vi "Subtract Resources (SubVI).vi"(8 "error in (no error)":errorcluster, 10 "Simulation in":cluster{"Water":dbl, "Coffee":dbl, "Milk":dbl}, 11 "Coffee Selection":T1) -> (0 "error out":errorcluster, 2 "Simulation out":cluster{"Water":dbl, "Coffee":dbl, "Milk":dbl}, 3 "Coffe and Chamber increase":cluster{"coffee":i8, "chamber":i8})   [LabVIEW 2017]
panel:
  # "input values"
  # "output values"
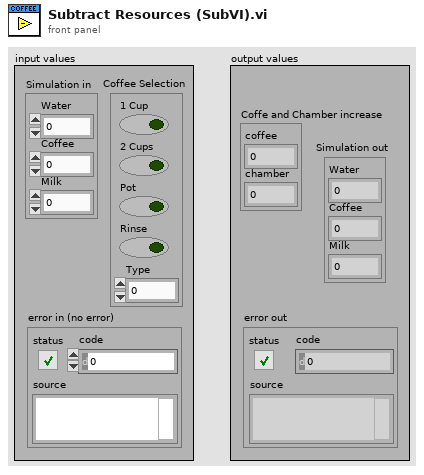
[diagram p1: front panel]
types:
  T1 = cluster{"1 Cup":bool, "2 Cups":bool, "Pot":bool, "Rinse":bool, "Type":i8}
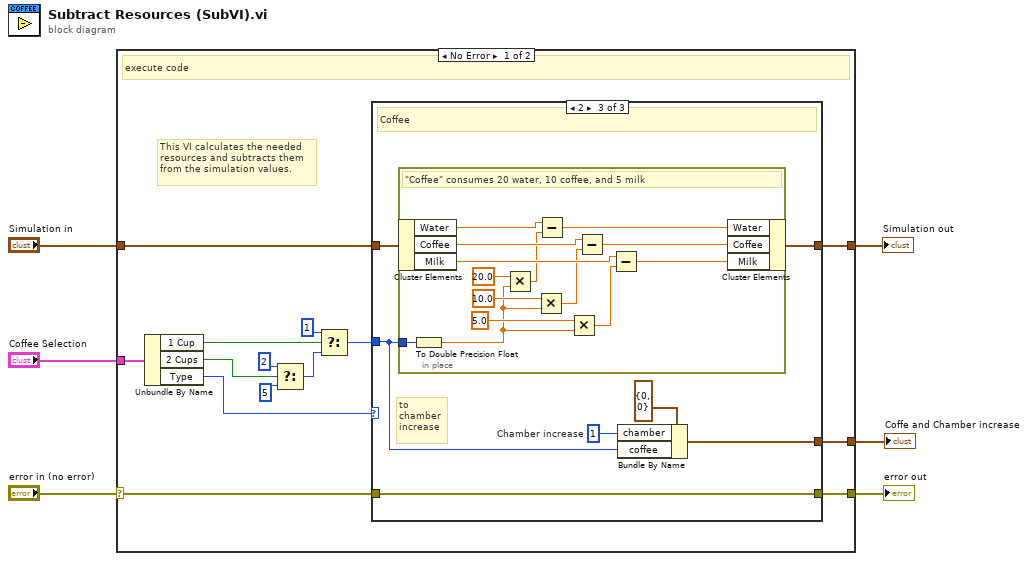
[diagram p0: block diagram]
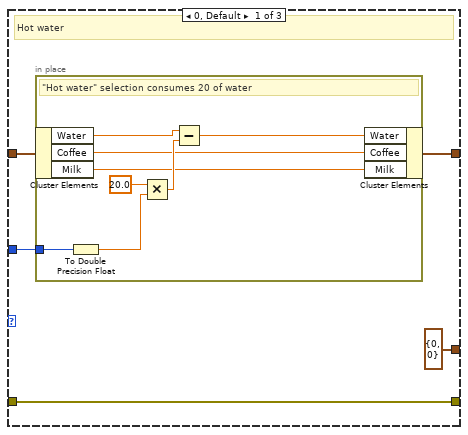
[diagram p2: hidden frame]
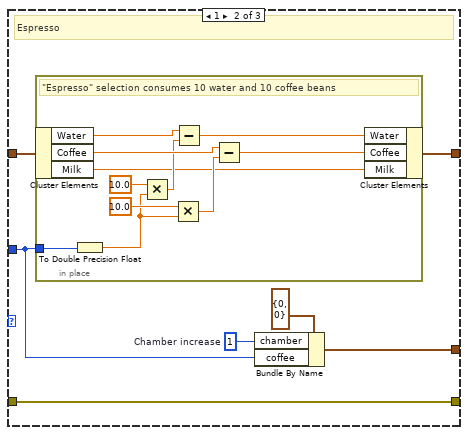
[diagram p3: hidden frame]
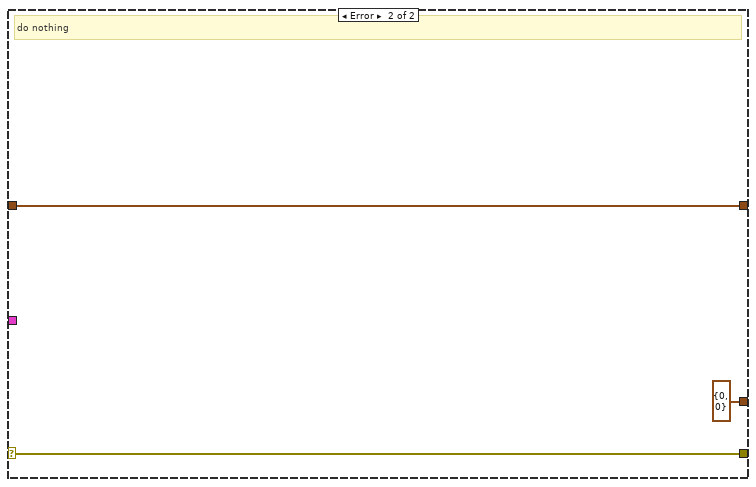
[diagram p4: hidden frame]
diagram:
  n1 = case shown="No Error" "error in (no error)" {
    selector: "error in (no error)" -> [w17 w74]
    tunnel: "Simulation in" -> [w20 w75]
    tunnel: "Coffee Selection" -> [w19 _]
    tunnel: [w18 w75] -> w4
    tunnel: [w16 w74] -> w2
    tunnel: [w15 cluster{"coffee":i8, "chamber":i8} {"coffee"=0, "chamber"=0} ("input cluster")] -> w1
    frame No Error {
      # "This VI calculates the needed\nresources and subtracts them\nfrom the simulation values."
      # "execute code"
      n2 = Unbundle By Name(w19) -> ("1 Cup"=w14:bool, "2 Cups"=w11:bool, "Type"=w10:i8)
      n3 = Select(t=i8 2, s=w11, f=i8 5) -> (s? t:f=w8:i8)
      n4 = Select(t=i8 1, s=w14, f=w8) -> (s? t:f=w13:i8)
      n5 = case shown="2" w10 {
        tunnel: w20 -> [w25 w40 w58]
        tunnel: [w24 w39 w57] -> w18
        tunnel: w13 -> [w23 w35 w53]
        tunnel: w17 -> [w22 w38 w56]
        tunnel: [w22 w38 w56] -> w16
        tunnel: [cluster{"coffee":i8, "chamber":i8} {"coffee"=0, "chamber"=0} ("input cluster") w37 w55] -> w15
        frame 0, Default {
          # "Hot water"
          n6 = in-place {
            in-place-border: w23 -> [w27]
            # "\"Hot water\" selection consumes 20 of water"
            n7 = in-place-cluster #1(w25) -> ("Water"=w33:dbl, "Coffee"=w29:dbl, "Milk"=w28:dbl)
            n8 = To Double Precision Float(number=w27) -> (double precision float=w26:dbl)
            n9 = Multiply(x=20.0, y=w26) -> (x*y=w30:dbl)
            n10 = Subtract(x=w33, y=w30) -> (x-y=w32:dbl)
            n11 = in-place-cluster #1("Water"=w32, "Coffee"=w29, "Milk"=w28) -> (w24:cluster{"Water":dbl, "Coffee":dbl, "Milk":dbl})
          }
        }
        frame 1 {
          w36 = i8 1  # Chamber increase
          # "Espresso"
          n12 = in-place {
            in-place-border: w35 -> [w42]
            # "\"Espresso\" selection consumes 10 water and 10 coffee beans"
            n13 = in-place-cluster #2(w40) -> ("Water"=w51:dbl, "Coffee"=w49:dbl, "Milk"=w43:dbl)
            n14 = To Double Precision Float(number=w42) -> (double precision float=w41:dbl)
            n15 = Multiply(x=10.0, y=w41) -> (x*y=w45:dbl)
            n16 = Multiply(x=10.0, y=w41) -> (x*y=w44:dbl)
            n17 = Subtract(x=w51, y=w45) -> (x-y=w50:dbl)
            n18 = Subtract(x=w49, y=w44) -> (x-y=w48:dbl)
            n19 = in-place-cluster #2("Water"=w50, "Coffee"=w48, "Milk"=w43) -> (w39:cluster{"Water":dbl, "Coffee":dbl, "Milk":dbl})
          }
          n20 = Bundle By Name(cluster=cluster{"coffee":i8, "chamber":i8} {"coffee"=0, "chamber"=0} ("output cluster"), "chamber"=w36, "coffee"=w35) -> (w37:cluster{"coffee":i8, "chamber":i8})
        }
        frame 2 {
          w54 = i8 1  # Chamber increase
          # "to\nchamber\nincrease"
          # "Coffee"
          n21 = in-place {
            in-place-border: w53 -> [w60]
            # "\"Coffee\" consumes 20 water, 10 coffee, and 5 milk"
            n22 = in-place-cluster #3(w58) -> ("Water"=w72:dbl, "Coffee"=w70:dbl, "Milk"=w68:dbl)
            n23 = To Double Precision Float(number=w60) -> (double precision float=w59:dbl)
            n24 = Multiply(x=20.0, y=w59) -> (x*y=w63:dbl)
            n25 = Multiply(x=10.0, y=w59) -> (x*y=w62:dbl)
            n26 = Subtract(x=w72, y=w63) -> (x-y=w71:dbl)
            n27 = Multiply(x=5.0, y=w59) -> (x*y=w61:dbl)
            n28 = Subtract(x=w70, y=w62) -> (x-y=w69:dbl)
            n29 = Subtract(x=w68, y=w61) -> (x-y=w67:dbl)
            n30 = in-place-cluster #3("Water"=w71, "Coffee"=w69, "Milk"=w67) -> (w57:cluster{"Water":dbl, "Coffee":dbl, "Milk":dbl})
          }
          n31 = Bundle By Name(cluster=cluster{"coffee":i8, "chamber":i8} {"coffee"=0, "chamber"=0} ("output cluster"), "chamber"=w54, "coffee"=w53) -> (w55:cluster{"coffee":i8, "chamber":i8})
        }
      }
    }
    frame Error {
      # "do nothing"
    }
  }
  "Simulation out" <- w4
  "error out" <- w2
  "Coffe and Chamber increase" <- w1
